vi "Gen - Filter Diff Array Item.vi"(7 "All Element":string[](array[string]), 11 "List in":string[](array[string])) -> (3 "List Out":string[](array[string]))   [LabVIEW 2020]
doc: "This VI used to remove a different element from array"
uses:
  13e3e3a5-2ae6-46b4-b79c-61b885b60aa3.vi
  <vilib>/Comparison/Equal/Equal Functor/Equal Functor.lvclass
panel:
  out "Error Out":errorcluster
  in  "Error In":errorcluster
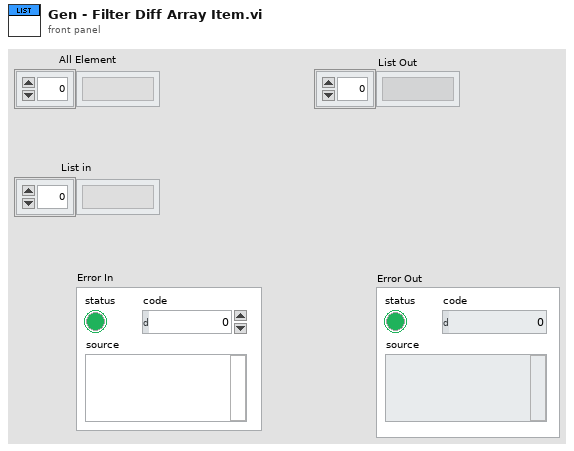
[diagram p1: front panel]
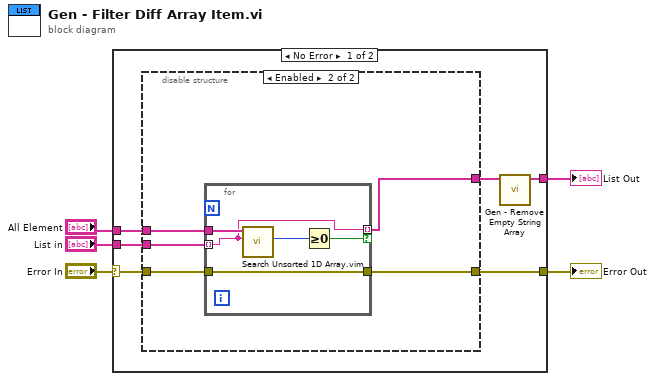
[diagram p0: block diagram]
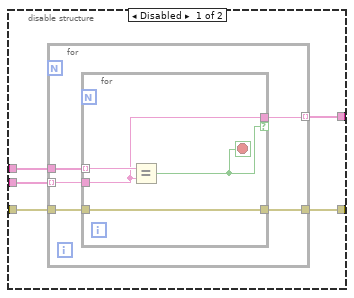
[diagram p2: hidden frame]
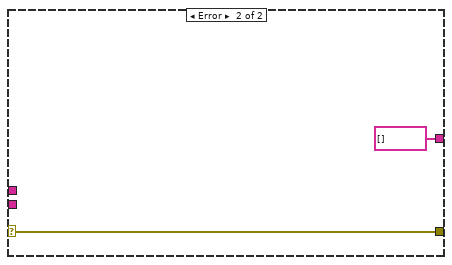
[diagram p3: hidden frame]
diagram:
  n1 = case shown="No Error" "Error In" {
    selector: "Error In" -> [w9 w37]
    tunnel: [w8 w37] -> w4
    tunnel: "All Element" -> [w11 _]
    tunnel: "List in" -> [w10 _]
    tunnel: [w6 string[] []] -> w3
    frame No Error {
      n2 = disable-structure shown="Enabled" {
        disable-tunnel: w11 -> [w16 w30]
        disable-tunnel: w10 -> [w15 w29]
        disable-tunnel: w9 -> [w14 w27]
        disable-tunnel: [w13 w26] -> w8
        disable-tunnel: [w12 w28] -> w7
        frame Disabled {
          n3 = for {
            tunnel: w16 -> [w21]
            tunnel: w15 -> [w20] mode=indexing
            tunnel: [w19] -> w12 mode=indexing
            tunnel: w14 -> [w18]
            tunnel: [w17] -> w13
            n4 = for {
              tunnel: w21 -> [w25] mode=indexing
              tunnel: w20 -> [w24]
              tunnel: [w24] -> w19 if=w23
              tunnel: w18 -> [w22]
              tunnel: [w22] -> w17
              stop <- w23 stop-if-true
              n5 = Equal?(x=w25, y=w24) -> (x = y?=w23:bool)
            }
          }
        }
        frame Enabled {
          n6 = for {
            tunnel: w30 -> [w35]
            tunnel: w29 -> [w33] mode=indexing
            tunnel: [w33] -> w28 mode=indexing if=w32
            tunnel: w27 -> [w31]
            tunnel: [w31] -> w26
            n7 = call "Search Unsorted 1D Array.vim"("element"=w33, "unsorted 1D array"=w35) -> ("index of element"=w34:i32)  [unwired: 9 in]
            n8 = Greater Or Equal To 0?(x=w34) -> (x >= 0?=w32:bool)
          }
        }
      }
      n9 = call "Gen - Remove Empty String Array.vi"("Data Array"=w7) -> ("Data Out"=w6:string[])  [unwired: 10 in]
    }
    frame Error {
    }
  }
  "Error Out" <- w4
  "List Out" <- w3
